vi "MB Serial Slave Demon.vi"(6 "Period":u32=200, 7 "Slave Address":u8 format="%.0x", 9 "Timeouts":u32[](array[numeric]), 10 "Modes":enum16{"RTU", "ASCII"}[](array[ring]), 11 "VISA Sessions":refnum<visa-resource-name>[](array[refnum])) -> ()   [LabVIEW 2023, in "Voegtlin_NI_SMART_Modbus_Drivers.lvlib"]
doc: "The serial slave demon constantly scans the serial port for commands from the master. When it detects a command from the master, it updates the memory tables with data and also responds to the master's query for data. You must use the slave API to access the data in the tables."
uses:
  Voegtlin_NI_SMART_Modbus_Drivers.lvlib
  MB RefCount Function.ctl
  MB Globals.vi
panel:
  in  "Case Constant\n(See Context Help)":bool
  out "Demon Running":bool
  # "VI Name: MB Serial Slave Demon.vi\nPurpose: Modbus Demon"
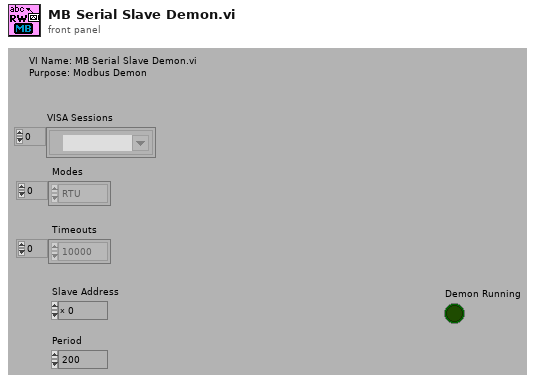
[diagram p1: front panel]
types:
  T1 = typedef "Voegtlin_NI_SMART_Modbus_Drivers.lvlib/MB RefCount Function.ctl" = enum16{"Init", "Add", "Remove", "Is Running?"}
  T2 = cluster{"Mode":enum16{"RTU", "ASCII"}, "Slave Address":u8}
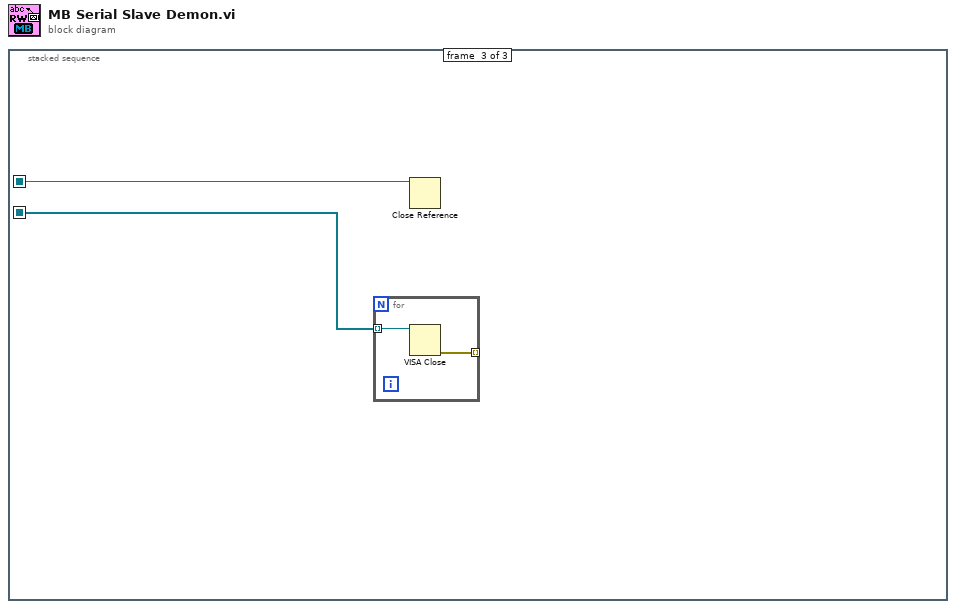
[diagram p0: block diagram]
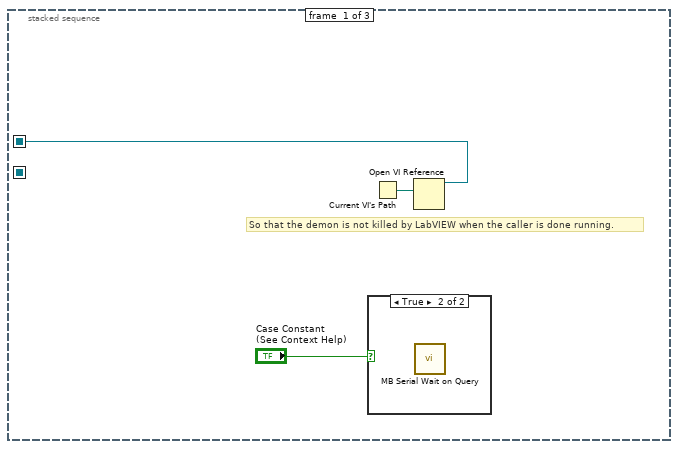
[diagram p2: hidden frame]
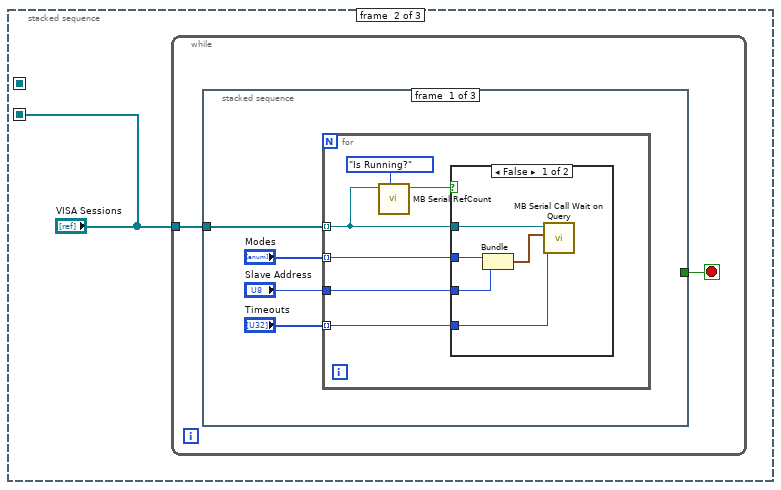
[diagram p4: hidden frame]
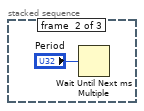
[diagram p6: hidden frame]
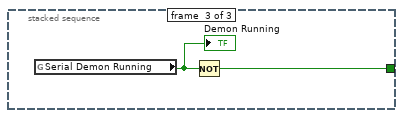
[diagram p7: hidden frame]
diagram:
  n1 = stacked-sequence {
    seq-local: [_ "VISA Sessions" _] -> [_ _ w26]
    seq-local: [w2 _ _] -> [_ _ w25]
    frame #0 {
      # "So that the demon is not killed by LabVIEW when the caller is done running."
      n2 = case shown="True" "Case Constant\n(See Context Help)" {
        frame False {
        }
        frame True {
          n3 = call "MB Serial Wait on Query.vi"() -> ()  [unwired: 1 in, 11 out]
        }
      }
      n4 = Current VI's Path() -> (path=w3:path)
      n5 = Open VI Reference(vi path=w3) -> (vi reference=w2:refnum<vi>)  [unwired: 1 in, 5 out]
    }
    frame #1 {
      n6 = while {
        tunnel: "VISA Sessions" -> [w6]
        stop <- w5 stop-if-true
        n7 = stacked-sequence {
          tunnel: w6 -> [w10 _ _]
          tunnel: [_ _ w23] -> w5
          frame #0 {
            n8 = for {
              tunnel: "Timeouts" -> [w16] mode=indexing
              tunnel: "Modes" -> [w15] mode=indexing
              tunnel: "Slave Address" -> [w14]
              tunnel: w10 -> [w12] mode=indexing
              n9 = call "MB Serial RefCount.vi"("Function"=MB_RefCount_Function."Is Running?", "VISA resource name"=w12) -> ("VI Running?"=w11:bool)  [unwired: 9 out]
              n10 = case shown="False" w11 {
                tunnel: w16 -> [w21 _]
                tunnel: w15 -> [w20 _]
                tunnel: w14 -> [w19 _]
                tunnel: w12 -> [w17 _]
                frame False {
                  n11 = Bundle("Mode"=w20, "Slave Address"=w19) -> (w18:T2)  [unwired: 1 out]
                  n12 = call "MB Serial Call Wait on Query.vi"("Timeout"=w21, "Serial Parameters"=w18, "VISA resource name"=w17) -> ()  [unwired: 9 out]
                }
                frame True {
                }
              }
            }
          }
          frame #1 {
            n13 = Wait Until Next ms Multiple(millisecond multiple="Period") -> ()  [unwired: 1 out]
          }
          frame #2 {
            n14 = global read "MB Globals.vi" "Serial Demon Running"() -> (w24:bool)
            "Demon Running" <- w24
            n15 = Not(x=w24) -> (.not. x?=w23:bool)
          }
        }
      }
    }
    frame #2 {
      n16 = for {
        tunnel: w26 -> [w28] mode=indexing
        tunnel: [w27] -> _ mode=indexing
        n17 = VISA Close(VISA resource name=w28) -> (error out=w27:errorcluster)  [unwired: 1 in]
      }
      n18 = Close Reference(reference=w25) -> ()  [unwired: 1 in, 1 out]
    }
  }
